vi "Main.vi"() -> ()   [LabVIEW 2018, in "Composite Pattern Demo.lvclass"]
uses:
  Composite Pattern Demo.lvclass
  Composite Employee Class/Composite Employee.lvclass
  ConsoleOut/Print Options.ctl
panel:
  out "error out":errorcluster
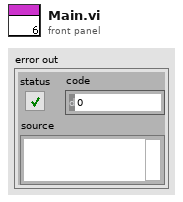
[diagram p1: front panel]
types:
  T1 = typedef "Print Options.ctl" = enum16{"Create", "Get Reference", "Print", "Print Header", "Close"}
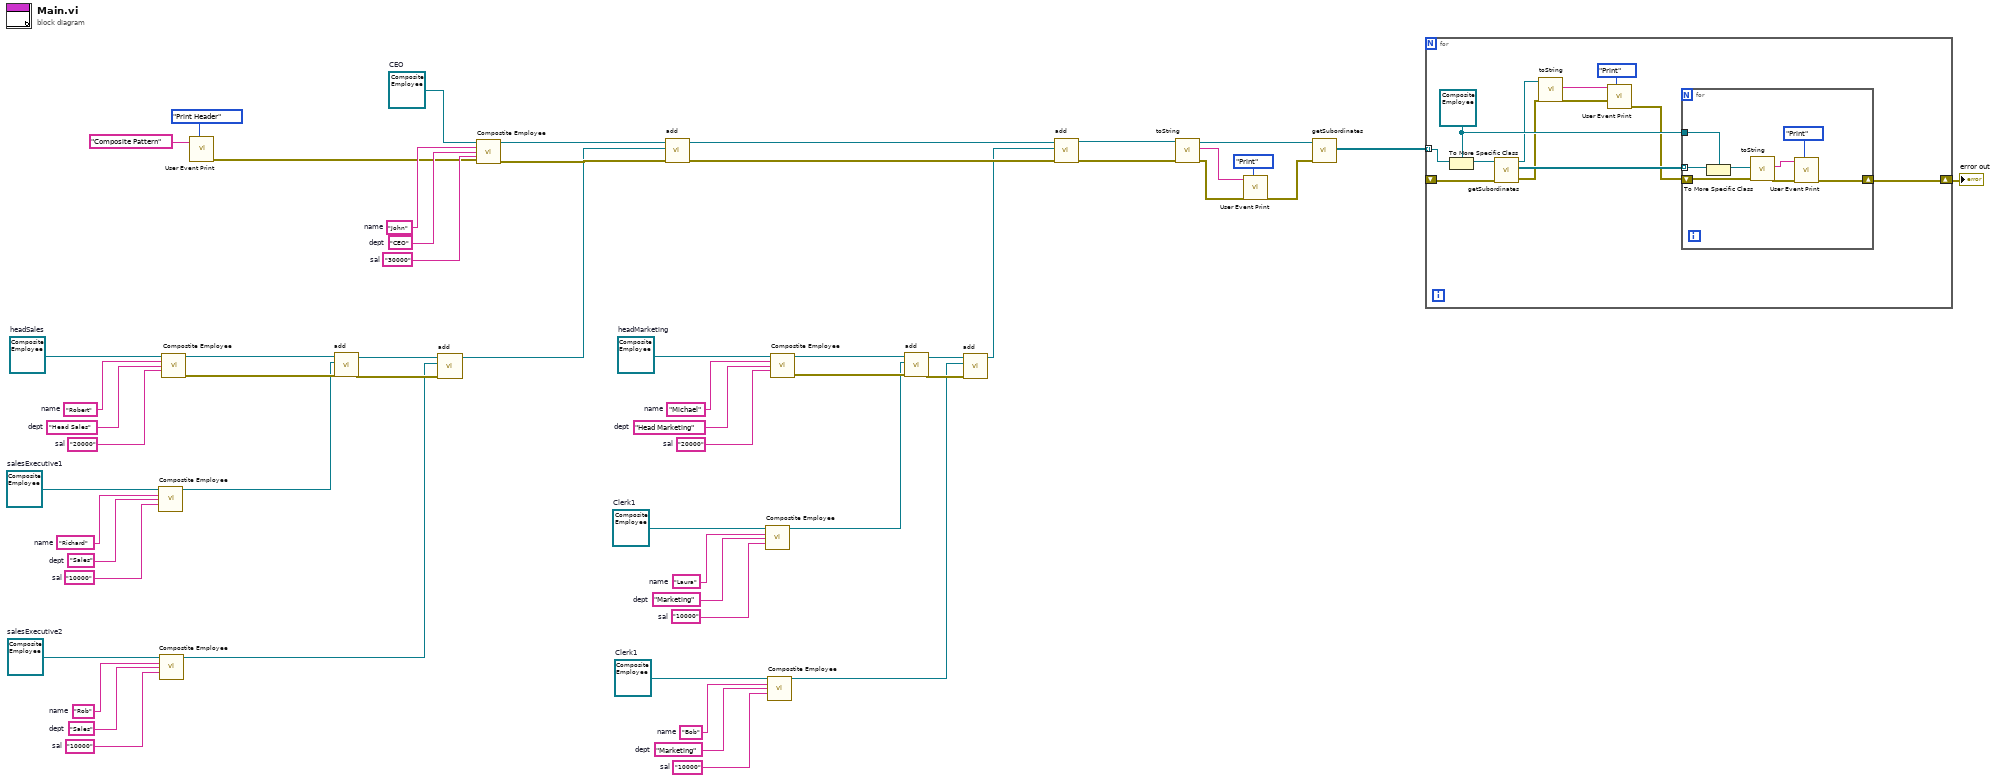
[diagram p0: block diagram]
diagram:
  w31 = "10000"  # sal
  w32 = "Sales"  # dept
  w33 = "Rob"  # name
  w34 = refnum<class "Composite Employee.lvclass"> refnum  # salesExecutive2
  w38 = "10000"  # sal
  w37 = "Sales"  # dept
  w36 = "Richard"  # name
  w35 = refnum<class "Composite Employee.lvclass"> refnum  # salesExecutive1
  w39 = "10000"  # sal
  w40 = "Marketing"  # dept
  w41 = "Bob"  # name
  w42 = refnum<class "Composite Employee.lvclass"> refnum  # Clerk1
  w46 = "10000"  # sal
  w45 = "Marketing"  # dept
  w44 = "Laura"  # name
  w43 = refnum<class "Composite Employee.lvclass"> refnum  # Clerk1
  w47 = "20000"  # sal
  w48 = "Head Marketing"  # dept
  w49 = "Michael"  # name
  w50 = refnum<class "Composite Employee.lvclass"> refnum  # headMarketing
  w54 = "20000"  # sal
  w53 = "Head Sales"  # dept
  w52 = "Robert"  # name
  w51 = refnum<class "Composite Employee.lvclass"> refnum  # headSales
  w55 = "30000"  # sal
  w56 = "CEO"  # dept
  w57 = "John"  # name
  w58 = refnum<class "Composite Employee.lvclass"> refnum  # CEO
  n1 = call-dynamic "Compostite Employee.vi"("Composite Employee in"=w35, "name"=w36, "dept"=w37, "sal"=w38) -> ("Composite Employee out"=w22:refnum<class "Composite Employee.lvclass">)  [unwired: 10 in, 1 out]
  n2 = call-dynamic "Compostite Employee.vi"("Composite Employee in"=w34, "name"=w33, "dept"=w32, "sal"=w31) -> ("Composite Employee out"=w21:refnum<class "Composite Employee.lvclass">)  [unwired: 10 in, 1 out]
  n3 = call-dynamic "Compostite Employee.vi"("Composite Employee in"=w51, "name"=w52, "dept"=w53, "sal"=w54) -> ("Composite Employee out"=w24:refnum<class "Composite Employee.lvclass">, "error out"=w23:errorcluster)  [unwired: 10 in]
  n4 = call "User Event Print.vi"("Options"=Print_Options."Print Header", "String to Print"="Composite Pattern") -> ("error out"=w5:errorcluster)  [unwired: 8 in, 1 out]
  n5 = call-dynamic "add.vi"("error in (no error)"=w23, "Composite Employee.lvclass"=w22, "Composite Employee in"=w24) -> ("error out"=w25:errorcluster, "Composite Employee out"=w26:refnum<class "Composite Employee.lvclass">)  [unwired: 7 in]
  n6 = call-dynamic "add.vi"("error in (no error)"=w25, "Composite Employee.lvclass"=w21, "Composite Employee in"=w26) -> ("Composite Employee out"=w20:refnum<class "Composite Employee.lvclass">)  [unwired: 7 in, 1 out]
  n7 = call-dynamic "Compostite Employee.vi"("Composite Employee in"=w58, "name"=w57, "dept"=w56, "sal"=w55, "error in (no error)"=w5) -> ("Composite Employee out"=w28:refnum<class "Composite Employee.lvclass">, "error out"=w27:errorcluster)  [unwired: 9 in]
  n8 = call-dynamic "add.vi"("error in (no error)"=w27, "Composite Employee.lvclass"=w20, "Composite Employee in"=w28) -> ("error out"=w29:errorcluster, "Composite Employee out"=w30:refnum<class "Composite Employee.lvclass">)  [unwired: 7 in]
  n9 = call-dynamic "Compostite Employee.vi"("Composite Employee in"=w43, "name"=w44, "dept"=w45, "sal"=w46) -> ("Composite Employee out"=w15:refnum<class "Composite Employee.lvclass">)  [unwired: 10 in, 1 out]
  n10 = call-dynamic "Compostite Employee.vi"("Composite Employee in"=w42, "name"=w41, "dept"=w40, "sal"=w39) -> ("Composite Employee out"=w14:refnum<class "Composite Employee.lvclass">)  [unwired: 10 in, 1 out]
  n11 = call-dynamic "Compostite Employee.vi"("Composite Employee in"=w50, "name"=w49, "dept"=w48, "sal"=w47) -> ("Composite Employee out"=w19:refnum<class "Composite Employee.lvclass">, "error out"=w18:errorcluster)  [unwired: 10 in]
  n12 = call-dynamic "add.vi"("error in (no error)"=w18, "Composite Employee.lvclass"=w15, "Composite Employee in"=w19) -> ("error out"=w16:errorcluster, "Composite Employee out"=w17:refnum<class "Composite Employee.lvclass">)  [unwired: 7 in]
  n13 = call-dynamic "add.vi"("error in (no error)"=w16, "Composite Employee.lvclass"=w14, "Composite Employee in"=w17) -> ("Composite Employee out"=w13:refnum<class "Composite Employee.lvclass">)  [unwired: 7 in, 1 out]
  n14 = call-dynamic "add.vi"("error in (no error)"=w29, "Composite Employee.lvclass"=w13, "Composite Employee in"=w30) -> ("error out"=w11:errorcluster, "Composite Employee out"=w12:refnum<class "Composite Employee.lvclass">)  [unwired: 7 in]
  n15 = call-dynamic "toString.vi"("error in (no error)"=w11, "Composite Employee in"=w12) -> ("error out"=w9:errorcluster, "resulting string"=w3:string, "Composite Employee out"=w10:refnum<class "Composite Employee.lvclass">)  [unwired: 7 in]
  n16 = call "User Event Print.vi"("Options"=Print_Options."Print", "error in (no error)"=w9, "String to Print"=w3) -> ("error out"=w4:errorcluster)  [unwired: 7 in, 1 out]
  n17 = call-dynamic "getSubordinates.vi"("error in (no error)"=w4, "Composite Employee in"=w10) -> ("subordinates"=w8:refnum<class "Employee.lvclass">[])  [unwired: 7 in, 2 out]
  n18 = for {
    tunnel: w8 -> [w70] mode=indexing
    shift-right: [w60] -> w1
    shift-left: _ -> [w59]
    w67 = refnum<class "Composite Employee.lvclass"> refnum ("Composite Employee.lvclass")
    n19 = To More Specific Class(target class=w67, reference=w70) -> (specific class reference=w69:refnum<class "Composite Employee.lvclass">)  [unwired: 1 in, 1 out]
    n20 = call-dynamic "getSubordinates.vi"("error in (no error)"=w59, "Composite Employee in"=w69) -> ("error out"=w62:errorcluster, "subordinates"=w68:refnum<class "Employee.lvclass">[], "Composite Employee out"=w66:refnum<class "Composite Employee.lvclass">)  [unwired: 7 in]
    n21 = call-dynamic "toString.vi"("error in (no error)"=w62, "Composite Employee in"=w66) -> ("error out"=w63:errorcluster, "resulting string"=w64:string)  [unwired: 7 in, 1 out]
    n22 = call "User Event Print.vi"("Options"=Print_Options."Print", "error in (no error)"=w63, "String to Print"=w64) -> ("error out"=w61:errorcluster)  [unwired: 7 in, 1 out]
    n23 = for {
      tunnel: w68 -> [w78] mode=indexing
      tunnel: w67 -> [w74]
      shift-right: [w73] -> w60
      shift-left: w61 -> [w76]
      n24 = To More Specific Class(target class=w74, reference=w78) -> (specific class reference=w77:refnum<class "Composite Employee.lvclass">)  [unwired: 1 in, 1 out]
      n25 = call-dynamic "toString.vi"("error in (no error)"=w76, "Composite Employee in"=w77) -> ("error out"=w75:errorcluster, "resulting string"=w72:string)  [unwired: 7 in, 1 out]
      n26 = call "User Event Print.vi"("Options"=Print_Options."Print", "error in (no error)"=w75, "String to Print"=w72) -> ("error out"=w73:errorcluster)  [unwired: 7 in, 1 out]
    }
  }
  "error out" <- w1
